vi "FlexRIOnoModule.vi"() -> ()   [LabVIEW 2013]
uses:
  Control 1.ctl
  ctl.ctl
  <vilib>/Platform/TimedLoop/XDataNode/timing_clust.ctl
  <vilib>/Platform/TimedLoop/XDataNode/nitl_modes.ctl
  <vilib>/Platform/TimedLoop/XDataNode/wakeup.ctl
  Libraries/StateControl.ctl
  Libraries/FlexRIO-NoModule/N Channels.ctl
  <vilib>/rvi/Emulation/niFpgaSctlEmulationGetInTimedLoop.vi
  <vilib>/rvi/Emulation/niFpgaEmulationReportErrorSimple.vi
  <vilib>/rvi/Emulation/niFpgaGetClockAttributes.vi
  <vilib>/rvi/Emulation/niFpgaCriticalErrorInLSC.vi
  <vilib>/rvi/FIFO/Fifo_Resource/nirvififoEmulationClearFpgaImpl.vi
  <vilib>/rvi/DataTransferAndStorage/Container/Common/niFpgaContainerGetUniqueNameForEmu.vi
  Libraries/GlobalReg.vi
  <vilib>/rvi/DataTransferAndStorage/Container/Common/niFpgaContainerExecOnDevCompGetState.vi
  <vilib>/rvi/FIFO/Fifo_Resource/nirvififoEmulationGetNumberOfElementsToReadFpgaImpl.vi
  <vilib>/rvi/interface/RandomDataEmulation/nirviRandomDataFPGAFIFO.vi
  <vilib>/rvi/interface/RandomDataEmulation/niFpgaRandomDataHandleErrors.vi
  <vilib>/rvi/eio/common/nirviEmuReportErrorAndStop.vi
  <vilib>/rvi/FIFO/Fifo_Resource/nirvififoEmulationReadFpgaImpl.vi
  <vilib>/rvi/FIFO/Fifo_Resource/nirvififoEmulationWriteFpgaImpl.vi
  <vilib>/rvi/Emulation/niFpgaProcessEmulError.vi
  <vilib>/rvi/eio/common/nirviEmuTemplateMethod_errors.vi
  <vilib>/Platform/TimedLoop/XDataNode/XDataNode.xnode
  <vilib>/rvi/DataTransferAndStorage/Container/XNode/niFpgaContainer.xnode
  <vilib>/rvi/FIFO/Fifo_Resource/nirvififoEmulationClear.vi
  <vilib>/rvi/FIFO/Fifo_Resource/niFpgaFifoEmulationRefIn.vi
  <vilib>/rvi/interface/RandomDataEmulation/nirviRandomDataFpgaReadWriteTemplate.vi
  <vilib>/eio/EIONode/EIONode.xnode
  <vilib>/rvi/FIFO/Fifo_Resource/nirvififoEmulationRead.vi
  <vilib>/Platform/TimedLoop/XDataNode/XDNodeRunTimeDep.lvlib
panel:
  in  "Cluster in":T1
  in  "Tab Control":T2(tab)=enum."Data Acquisition"
  out "Platform":enum8{"FlexRIO", "cRIO", "RSeries"}(ring)
  out "FPGAVIversion":u8[](array[numeric])=[1, 1]
  out "InitDone":bool
  out "RIOAdapterCorrect":bool
  out "Fref":u32=100000000
  out "DevQualityStatus":u8
  out "DevTemp":i16=-10244
  out "DevProfile":u8 format="%x"
  in  "DAQStartStop":bool
  in  "DebugMode":bool
  out "Expected IO Module ID":u32 format="%x"
  out "InsertedIOModule ID":u32
  out "DMATtoHOSTNCh":T3[](array[typedef])=[4]
  out "DMATtoHOSTFrameType":u8[](array[numeric])
  out "DMATtoHOSTSampleSize":u8[](array[numeric])=[2]
  out "DMATtoHOSTBlockNWords":u16[](array[numeric])=[4096]
  in  "DMATtoHOSTSamplingRate0":u16=10000
  in  "DMATtoHOSTEnable0":bool
  out "DMATtoHOSTOverflows":u16
  out "auxAI5":i32
  out "auxAI4":i32
  out "auxAI3":i32
  out "auxAI2":i32
  out "auxAI1":i32
  out "auxAI0":i32
  out "auxAI6":i32
  out "auxAI7":i32
  out "auxAI8":i32
  in  "auxAO5":i32
  in  "auxAO4":i32
  in  "auxAO3":i32
  in  "auxAO2":i32
  in  "auxAO1":i32
  in  "auxAO0":i32
  out "auxDI5":bool
  out "auxDI4":bool
  out "auxDI3":bool
  out "auxDI2":bool
  out "auxDI1":bool
  out "auxDI0":bool
  in  "auxDO3":bool
  in  "auxDO4":bool
  in  "auxDO5":bool
  in  "auxDO2":bool
  in  "auxDO1":bool
  in  "auxDO0":bool
  in  "AOEnable0":bool
  in  "SGUpdateRate0":u32=40
  in  "SGSignalType0":u8
  in  "SGPhase0":u32
  in  "SGFreq0":u32=100000
  in  "SGAmp0":u16
  in  "AO0":i32
  out "auxAI9":i32
  out "SGNo":u8=1 format="%x"
  out "SGFref0":u32=100000000
  # "Inputs"
  # "Aux Analog Input"
  # "Aux Digital Input"
  # "Outputs"
  # "Analog Output"
  # "Number of WF gen"
  # "Signal Generator 0"
  # "Aux Digital Output"
  # "Aux Analog Output"
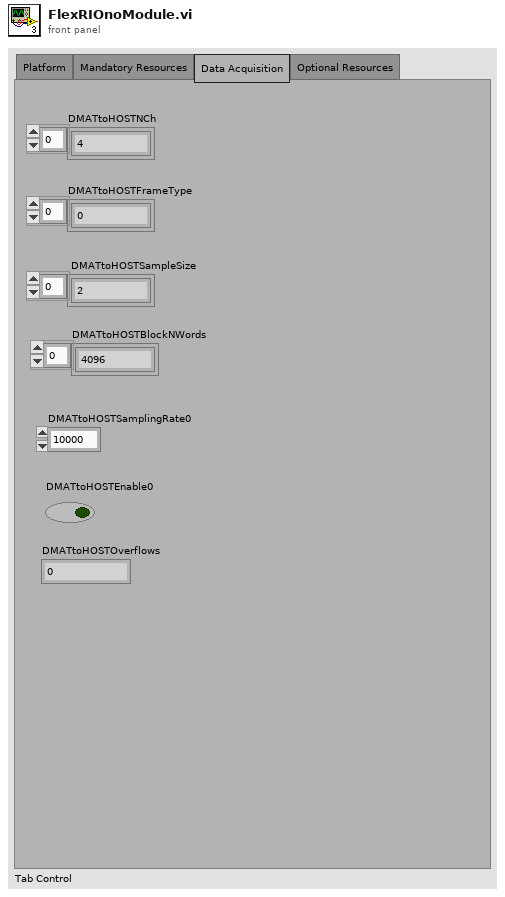
[diagram p1: front panel]
types:
  T1 = typedef "ctl.ctl" = cluster{"Number of sample in a block (0-4095)":u16, "SamplingRateN (Default 5000) (Decimation factor from ref clock)":u16, "Channels shif register up to 4 (A) ":u64, "Channels shif register up to 4 (B) ":u64, "Channels shif register up to 4 (C) ":u64, "Info shift register":u64, "ramp counter":i16, "GroupEnableN":bool, "Debug activation":bool, "Sample counter ":u64, "Decimation counter":u16, "Blocks counter":u16}
  T2 = enum32{"Platform", "Mandatory Resources", "Data Acquisition", "Optional Resources"}
  T3 = typedef "Control 1.ctl" = u16
  T4 = typedef "XDNodeRunTimeDep.lvlib/timing_clust.ctl" = cluster{"Expected End [f-1]":u64, "Actual End [f-1]":u64, "Finished Late? [f-1]":bool, "Expected End [i-1]":u64, "Actual End [i-1]":u64, "Finished Late? [i-1]":bool, "Expected Start [i]":u64, "Actual Start [i]":u64, "Expected Start [f]":u64, "Actual Start [f]":u64, "Source Name":string, "Structure Name":string, "Period":i64, "Deadline":i64, "Offset":i64, "Start":i64, "Priority":i32, "Timeout":i32, "Mode":T5, "Wakeup Reason":T6, "Error":errorcluster, "Source Type":string, "Secondary Source Type":string, "Global End Time":u64, "Global Start Time":u64, "Frame Duration":u64, "Iteration Duration":u64, "Assigned CPU":i32, "I/O Scan Engine Mode":u32}
  T5 = typedef "XDNodeRunTimeDep.lvlib/nitl_modes.ctl" = enum32{"No Change", "Process missed periods, maintain original phase", "Discard missed periods, maintain original phase", "Process missed periods, ignore original phase", "Discard missed periods, ignore original phase"}
  T6 = typedef "XDNodeRunTimeDep.lvlib/wakeup.ctl" = enum32{"Normal", "Aborted", "Asynchronous wakeup", "Timing source error", "Timed loop error", "Timeout"}
  T7 = typedef "StateControl.ctl" = enum16{"Idle", "Acq"}
  T8 = typedef "N Channels.ctl" = enum16{"0 Channels", "1 Channels", "2 Channels", "3 Channels", "4 Channels", "5 Channels", "6 Channels", "7 Channels", "8 Channels", "9 Channels", "10 Channels", "11 Channels", "12 Channels"}
  T9 = cluster{u16, u16, u64, u64, u64, u64, i16, bool, bool, u64, u16, u16}
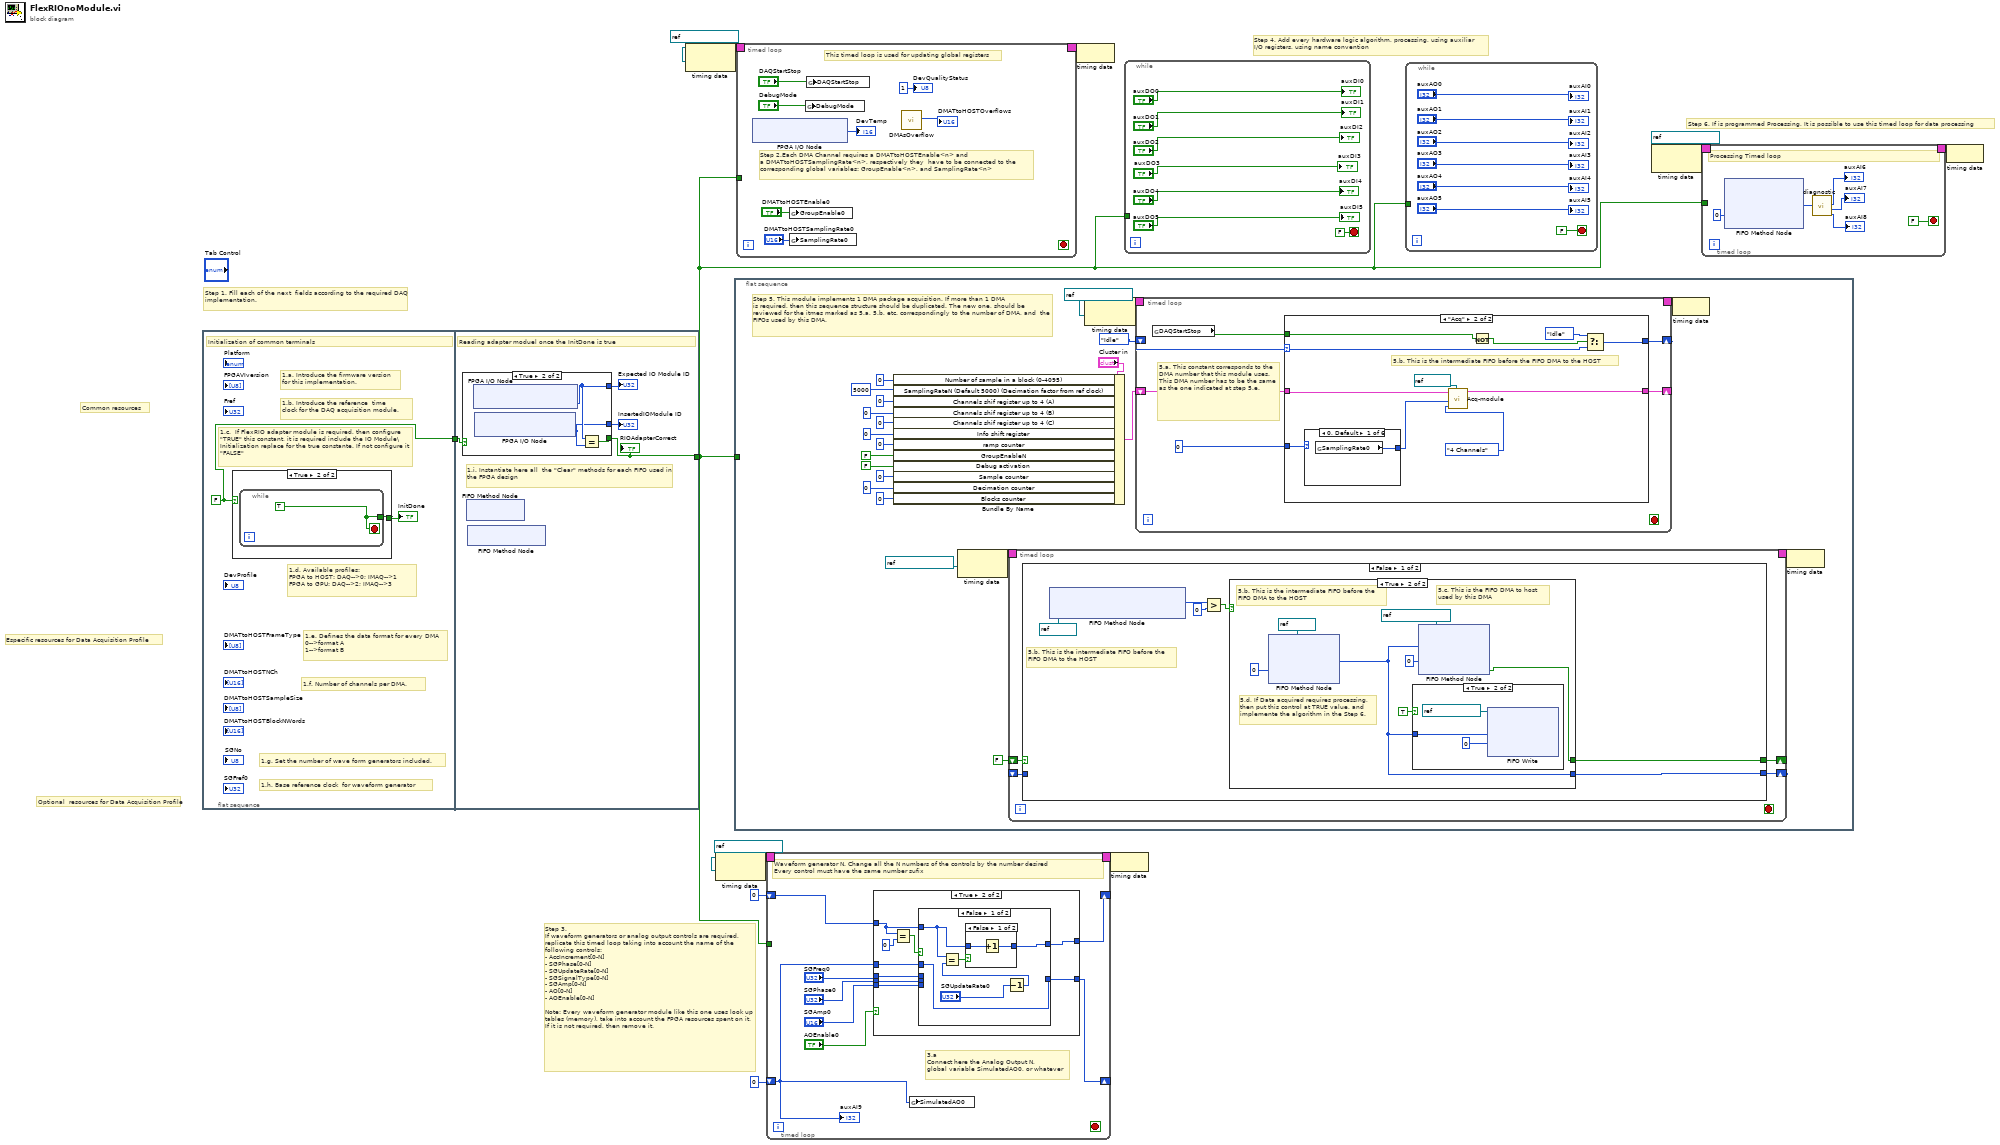
[diagram p0: block diagram]
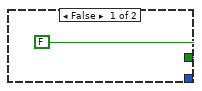
[diagram p2: hidden frame]
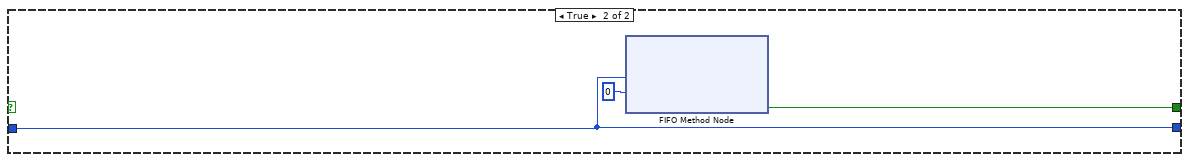
[diagram p4: hidden frame]
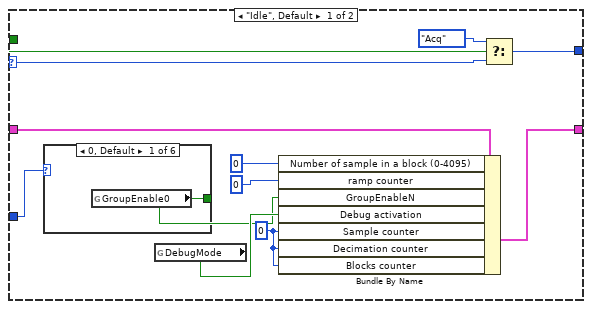
[diagram p5: hidden frame]
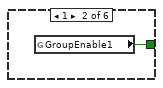
[diagram p6: hidden frame]
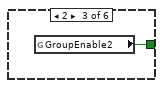
[diagram p7: hidden frame]
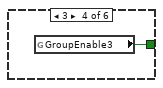
[diagram p8: hidden frame]
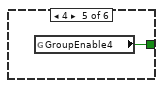
[diagram p9: hidden frame]
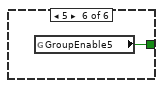
[diagram p10: hidden frame]
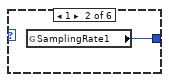
[diagram p11: hidden frame]
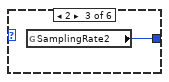
[diagram p12: hidden frame]
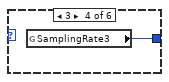
[diagram p13: hidden frame]
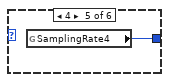
[diagram p14: hidden frame]
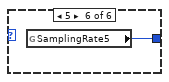
[diagram p15: hidden frame]
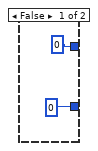
[diagram p16: hidden frame]
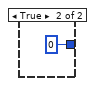
[diagram p17: hidden frame]
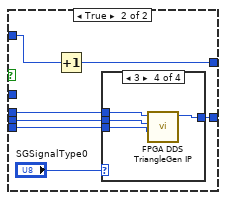
[diagram p18: hidden frame]
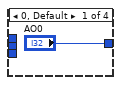
[diagram p19: hidden frame]
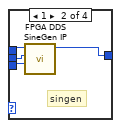
[diagram p20: hidden frame]
diagram:
  # "Optional  resources for Data Acquisition Profile"
  # "Especific resources for Data Acquisition Profile"
  # "Common resources"
  # "Step 6. If is programmed Processing, It is possible to use this timed loop for data processing"
  # "Step 4. Add every hardware logic algorithm, processing, using auxiliar \nI/O registers, using name convention"
  # "Step 3.\nIf waveform generators or analog output controls are required,\nreplicate this timed loop taking into account the name of the \nfollowing controls:\n- AccIncrement[0-N]\n- SGPhase[0-N]\n- SGUpdateRate[0-N]\n- SGSignalType[0-N]\n- SGAmp[0-N]\n- AO[0-N]\n- AOEnable[0-N]\n\nNote: Every waveform generator module like this one uses look up tables (memory), take into account the FPGA resources spent on it.  If it is not required, then remove it."
  # "Step 1. Fill each of the next  fields according to the required DAQ implementation."
  n1 = flat-sequence {
    tunnel: [w14] -> w13
    tunnel: [w21] -> w1
    tunnel: w13 -> [w20]
    frame #0 {
      w14 = FALSE
      # "1.h. Base reference clock  for waveform generator"
      # "1.e. Defines the data format for every DMA\n0-->format A\n1-->format B"
      # "1.c.  If FlexRIO adapter module is required, then configure \"TRUE\" this constant, it is required include the IO Module\\Initialization replace for the true constante. If not configure it \"FALSE\""
      # "1.a. Introduce the firmware version \nfor this implementation."
      # "1.b. Introduce the reference  time \nclock for the DAQ acquisition module."
      # "1.g. Set the number of wave form generators included."
      # "1.f. Number of channels per DMA."
      # "1.d. Available profiles: \nFPGA to HOST: DAQ-->0; IMAQ-->1\nFPGA to GPU: DAQ-->2; IMAQ-->3"
      # "Initialization of common terminals"
      n2 = case shown="True" w14 {
        tunnel: [w16 w18] -> w15
        frame False {
          n3 = while {
            tunnel: [w17] -> w16
            stop <- w17 stop-if-true
            w17 = TRUE
          }
        }
        frame True {
          n4 = while {
            tunnel: [w19] -> w18
            stop <- w19 stop-if-true
            w19 = TRUE
          }
        }
      }
      "InitDone" <- w15
    }
    frame #1 {
      # "1.i. Instantiate here all  the \"Clear\" methods for each FIFO used in the FPGA design"
      # "Reading adapter moduel once the InitDone is true"
      n5 = case shown="True" w20 {
        tunnel: [TRUE w28] -> w21
        tunnel: [w25 w27] -> w23
        tunnel: [w25 w26] -> w22
        frame False {
          w25 = u32 0
        }
        frame True {
          n6 = xnode "FPGA I/O Node"() -> ("Expected IO Module ID"=w27:u32)  [unwired: 1 in, 1 out]
          n7 = xnode "FPGA I/O Node"() -> ("Inserted IO Module ID"=w26:u32)  [unwired: 1 in, 1 out]
          n8 = Equal?(x=w27, y=w26) -> (x = y?=w28:bool)
        }
      }
      "Expected IO Module ID" <- w23
      "InsertedIOModule ID" <- w22
      "RIOAdapterCorrect" <- w21
      n9 = xnode ("FIFO Method Node")() -> ()  [unwired: 1 in, 1 out]
      n10 = xnode ("FIFO Method Node")() -> ()  [unwired: 1 in, 1 out]
    }
  }
  n11 = node-c288(refnum<k21> "100 MHz Clock" ("Source Name")) -> (w7:T4)
  n12 = node-c288(refnum<k21> "100 MHz Clock" ("Source Name")) -> (w12:T4)
  n13 = flat-sequence {
    tunnel: w1 -> [_]
    frame #0 {
      # "Step 5. This module implements 1 DMA package acquisition. If more than 1 DMA \nis required, then this sequence structure should be duplicated. The new one, should be \nreviewed for the itmes marked as 5.a, 5.b, etc. correspondingly to the number of DMA, and  the FIFOs used by this DMA."
      n14 = Bundle By Name(cluster="Cluster in", "Number of sample in a block (0-4095)"=u16 0 ("sample of block out"), "SamplingRateN (Default 5000) (Decimation factor from ref clock)"=u16 5000 ("FS1"), "Channels shif register up to 4 (A)"=u64 0, "Channels shif register up to 4 (B)"=u64 0, "Channels shif register up to 4 (C)"=u64 0, "Info shift register"=u64 0 ("Element"), "ramp counter"=i16 0, "GroupEnableN"=FALSE ("DMA1activation"), "Debug activation"=FALSE, "Sample counter"=u64 0 ("contador muestra"), "Decimation counter"=u16 0, "Blocks counter"=u16 0) -> (w31:T1)
      n15 = node-c288(refnum<k21> "100 MHz Clock" ("Source Name")) -> (w48:T4)
      n16 = timed-loop {
        timing: w48 -> [_]
        timing-out: [_] -> w47
        shift-right: [w54] -> _
        shift-left: FALSE ("Timed Out?") -> [w53]
        shift-right: [w52] -> _
        shift-left: _ -> [w51]
        stop <- _ stop-if-true
        n17 = case shown="False" w53 {
          tunnel: [w57 w73] -> w54
          tunnel: [w56 w72] -> w52
          tunnel: w51 -> [_ w72]
          frame False {
            # "5.b. This is the intermediate FIFO before the \nFIFO DMA to the HOST"
            n18 = xnode ("FIFO Method Node")("FIFO In"=refnum<k21> "FIFO0" ("IntermediateFIFO")) -> ("Number of Elements to Read"=w60:u32)  [unwired: 1 out]
            n19 = Greater?(x=w60, y=u32 0) -> (0:w58:bool)
            n20 = case shown="True" w58 {
              tunnel: [FALSE ("Timed Out?") w66] -> w57
              tunnel: [_ w65] -> w56
              frame False {
              }
              frame True {
                # "5.d. If Data acquired requires processing,\nthen put this control at TRUE value, and\nimplemente the algorithm in the Step 6."
                # "5.c. This is the FIFO DMA to host \nused by this DMA"
                # "5.b. This is the intermediate FIFO before the \nFIFO DMA to the HOST"
                n21 = xnode ("FIFO Method Node")("Timeout"=0, "FIFO In"=refnum<k21> "FIFO0" ("IntermediateFIFO")) -> ("Element"=w65:u64)  [unwired: 2 out]
                n22 = case shown="True" TRUE {
                  tunnel: w65 -> [_ w70]
                  frame False {
                  }
                  frame True {
                    n23 = xnode ("FIFO Write")("Element"=w70, "Timeout"=0, "FIFO In"=refnum<k21> "Processing0") -> ()  [unwired: 2 out]
                  }
                }
                n24 = xnode ("FIFO Method Node")("Element"=w65, "Timeout"=0, "FIFO In"=refnum<k21> "DMATtoHOST0") -> ("Timed Out?"=w66:bool)  [unwired: 1 out]
              }
            }
          }
          frame True {
            n25 = xnode ("FIFO Method Node")("Element"=w72, "Timeout"=0) -> ("Timed Out?"=w73:bool)  [unwired: 1 in, 1 out]
          }
        }
      }
      n26 = node-c288(refnum<k21> "100 MHz Clock" ("Source Name")) -> (w50:T4)
      n27 = timed-loop {
        timing: w50 -> [_]
        timing-out: [_] -> w49
        shift-right: [w85] -> _
        shift-left: StateControl."Idle" ("Enum") -> [w86]
        shift-right: [w82] -> _
        shift-left: w31 -> [w83]
        stop <- _ stop-if-true
        # "5.a. This constant corresponds to the DMA number that this module uses. This DMA number has to be the same as the one indicated at step 5.e."
        n28 = global read "GlobalReg.vi" "DAQStartStop"() -> (w84:bool)
        n29 = case shown="\"Acq\"" w86 {
          selector: w86 -> [w96 w114]
          tunnel: w84 -> [w98 w105]
          tunnel: [w95 w113] -> w85
          tunnel: w83 -> [w94 w111]
          tunnel: [w89 w110] -> w82
          tunnel: i16 0 ("DMA number") -> [w87 w107]
          frame "Idle", Default {
            w88 = i16 0
            n30 = case shown="0, Default" w87 {
              tunnel: [w99 w100 w101 w102 w103 w104] -> w90
              frame 0, Default {
                n31 = global read "GlobalReg.vi" "GroupEnable0"() -> (w99:bool)
              }
              frame 1 {
                n32 = global read "GlobalReg.vi" "GroupEnable1"() -> (w100:bool)
              }
              frame 2 {
                n33 = global read "GlobalReg.vi" "GroupEnable2"() -> (w101:bool)
              }
              frame 3 {
                n34 = global read "GlobalReg.vi" "GroupEnable3"() -> (w102:bool)
              }
              frame 4 {
                n35 = global read "GlobalReg.vi" "GroupEnable4"() -> (w103:bool)
              }
              frame 5 {
                n36 = global read "GlobalReg.vi" "GroupEnable5"() -> (w104:bool)
              }
            }
            n37 = global read "GlobalReg.vi" "DebugMode"() -> (w91:bool)
            n38 = Bundle By Name(cluster=w94, "Number of sample in a block (0-4095)"=u16 0, "ramp counter"=u64 0, "GroupEnableN"=w90, "Debug activation"=w91, "Sample counter"=w88, "Decimation counter"=w88, "Blocks counter"=w88) -> (w89:T1)
            n39 = Select(t=StateControl."Acq" ("Enum"), s=w98, f=w96) -> (s? t:f=w95:T7)
          }
          frame "Acq" {
            # "5.b. This is the intermediate FIFO before the FIFO DMA to the HOST"
            n40 = case shown="0, Default" w107 {
              tunnel: [w116 w117 w118 w119 w120 w121] -> w112
              frame 0, Default {
                n41 = global read "GlobalReg.vi" "SamplingRate0"() -> (w116:u16)
              }
              frame 1 {
                n42 = global read "GlobalReg.vi" "SamplingRate1"() -> (w117:u16)
              }
              frame 2 {
                n43 = global read "GlobalReg.vi" "SamplingRate2"() -> (w118:u16)
              }
              frame 3 {
                n44 = global read "GlobalReg.vi" "SamplingRate3"() -> (w119:u16)
              }
              frame 4 {
                n45 = global read "GlobalReg.vi" "SamplingRate4"() -> (w120:u16)
              }
              frame 5 {
                n46 = global read "GlobalReg.vi" "SamplingRate5"() -> (w121:u16)
              }
            }
            n47 = call "Acq-module.vi"("IntermediateFIFO"=refnum<k21> "FIFO0", "NumChannels"=N_Channels."4 Channels", "SamplingRate0"=w112, "Cluster in"=w111) -> ("cluster out"=w110:T9)  [unwired: 7 in]
            n48 = Not(x=w105) -> (.not. x?=w106:bool)
            n49 = Select(t=StateControl."Idle" ("Enum"), s=w106, f=w114) -> (s? t:f=w113:T7)
          }
        }
      }
      n50 = node-c288(w49) -> ()
      n51 = node-c288(w47) -> ()
    }
  }
  n52 = timed-loop {
    timing: w7 -> [_]
    timing-out: [_] -> w6
    tunnel: w1 -> [_]
    stop <- _ stop-if-true
    # "This timed loop is used for updating global registers"
    # "Step 2.Each DMA Channel requires a DMATtoHOSTEnable<n> and\na DMATtoHOSTSamplingRate<n>, respectively they  have to be connected to the\ncorresponding global variables: GroupEnable<n>, and SamplingRate<n>"
    n53 = xnode "FPGA I/O Node"() -> ("Device Temperature"=→"DevTemp":i16)  [unwired: 1 in, 1 out]
    n54 = global write "GlobalReg.vi" "GroupEnable0"("DMATtoHOSTEnable0") -> ()
    n55 = global write "GlobalReg.vi" "SamplingRate0"("DMATtoHOSTSamplingRate0") -> ()
    n56 = global write "GlobalReg.vi" "DebugMode"("DebugMode") -> ()
    n57 = global write "GlobalReg.vi" "DAQStartStop"("DAQStartStop") -> ()
    n58 = call "DMAsOverflow.vi"() -> ("DMAsOverFlow"=→"DMATtoHOSTOverflows":u16)  [unwired: 11 in]
    "DevQualityStatus" <- u8 1 ("DevQualityStatus")
  }
  n59 = timed-loop {
    shift-right: [w140] -> _
    shift-left: i16 0 ("Signal Value") -> [w137]
    timing: w12 -> [_]
    timing-out: [_] -> w11
    shift-right: [w138] -> _
    shift-left: u32 0 -> [w139]
    tunnel: w1 -> [_]
    stop <- _ stop-if-true
    # "3.a\nConnect here the Analog Output N,\nglobal variable SimulatedAO0, or whatever"
    # "Waveform generator N. Change all the N numbers of the controls by the number desired\nEvery control must have the same number sufix"
    n60 = case shown="True" "AOEnable0" {
      tunnel: "SGFreq0" -> [_ w155]
      tunnel: "SGPhase0" -> [_ w154]
      tunnel: "SGAmp0" -> [_ w153]
      tunnel: [i16 0 w152] -> w140
      tunnel: w139 -> [_ w149]
      tunnel: [u32 0 w148] -> w138
      tunnel: w137 -> [_ w147]
      frame False {
      }
      frame True {
        n61 = Equal?(x=w149, y=u32 0) -> (x = y?=w151:bool)
        n62 = case shown="False" w151 {
          tunnel: w155 -> [_ w171]
          tunnel: w154 -> [_ w170]
          tunnel: w153 -> [_ w169]
          tunnel: [w160 w168] -> w152
          tunnel: w149 -> [w159 w166]
          tunnel: [w161 w165] -> w148
          tunnel: w147 -> [w160 _]
          frame False {
            n63 = Decrement(x="SGUpdateRate0") -> (x-1=w157:u32)
            n64 = Equal?(x=w159, y=w157) -> (x = y?=w158:bool)
            n65 = case shown="False" w158 {
              tunnel: w159 -> [w163 _]
              tunnel: [w162 u32 0] -> w161
              frame False {
                n66 = Increment(x=w163) -> (x+1=w162:u32)
              }
              frame True {
              }
            }
          }
          frame True {
            n67 = Increment(x=w166) -> (x+1=w165:u32)
            n68 = case shown="3" "SGSignalType0" {
              tunnel: w171 -> [_ w176 w180 w184]
              tunnel: w170 -> [_ w175 w179 w183]
              tunnel: w169 -> [_ w174 w178 w182]
              tunnel: ["AO0" w173 w177 w181] -> w168
              frame 0, Default {
              }
              frame 1 {
                # "singen"
                n69 = call "FPGA DDS SineGen IP.vi"("Signal Amplitude (x 2^15)"=w174, "Phase Shift"=w175, "Accumulator Increment"=w176) -> ("Signal Value"=w173:i16)  [unwired: 7 in, 1 out]
              }
              frame 2 {
                # "square"
                n70 = call "FPGA DDS SquareGen IP.vi"("Signal Amplitude (x 2^15)"=w178, "Phase Shift"=w179, "Accumulator Increment"=w180) -> ("Signal Value"=w177:i16)  [unwired: 7 in, 1 out]
              }
              frame 3 {
                n71 = call "FPGA DDS TriangleGen IP.vi"("Signal Amplitude (x 2^15)"=w182, "Phase Shift"=w183, "Accumulator Increment"=w184) -> ("Signal Value"=w181:i16)  [unwired: 7 in, 1 out]
              }
            }
          }
        }
      }
    }
    n72 = global write "GlobalReg.vi" "SimulatedAO0"(w137) -> ()
    "auxAI9" <- w137
  }
  n73 = node-c288(w6) -> ()
  n74 = node-c288(w11) -> ()
  n75 = while {
    tunnel: w1 -> [_]
    stop <- FALSE stop-if-true
    "auxDI0" <- "auxDO0"
    "auxDI1" <- "auxDO1"
    "auxDI2" <- "auxDO2"
    "auxDI3" <- "auxDO3"
    "auxDI4" <- "auxDO4"
    "auxDI5" <- "auxDO5"
  }
  n76 = while {
    tunnel: w1 -> [_]
    stop <- FALSE stop-if-true
    "auxAI0" <- "auxAO0"
    "auxAI1" <- "auxAO1"
    "auxAI2" <- "auxAO2"
    "auxAI3" <- "auxAO3"
    "auxAI4" <- "auxAO4"
    "auxAI5" <- "auxAO5"
  }
  n77 = node-c288(refnum<k21> "100 MHz Clock" ("Source Name")) -> (w4:T4)
  n78 = timed-loop {
    timing: w4 -> [_]
    timing-out: [_] -> w3
    tunnel: w1 -> [_]
    stop <- FALSE stop-if-true
    # "Processing Timed loop"
    n79 = xnode ("FIFO Method Node")("Timeout"=0) -> ("Element"=w205:u64)  [unwired: 1 in, 2 out]
    n80 = call "diagnostic.vi"("Inp"=w205) -> ("diagnostic3"=→"auxAI8":i32, "diagnostic2"=→"auxAI7":i32, "diagnostic1"=→"auxAI6":i32)  [unwired: 8 in]
  }
  n81 = node-c288(w3) -> ()
